vi "Set up rotary stage.vi"(8 "error in (no error)":errorcluster, 11 "AOTF in":refnum<class "AOTF.lvclass">) -> (0 "error out":errorcluster, 3 "AOTF out":refnum<class "AOTF.lvclass">)   [LabVIEW 2012, in "AOTF.lvclass"]
uses:
  AOTF.lvclass
  AOTF.lvclass/AOTF.ctl
panel:
  in  "MG17Motor":refnum<k7>(container)
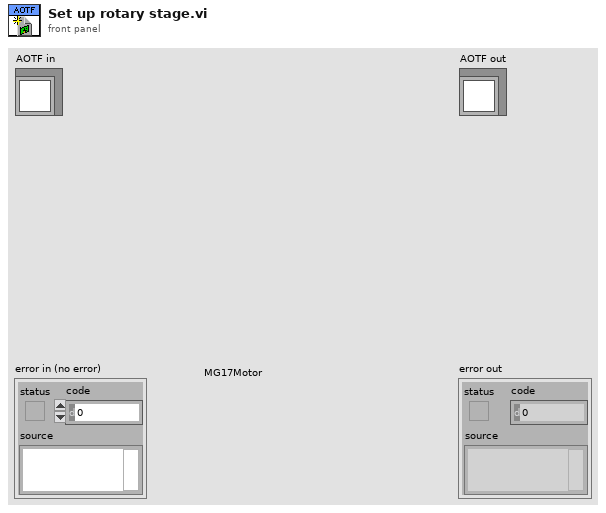
[diagram p1: front panel]
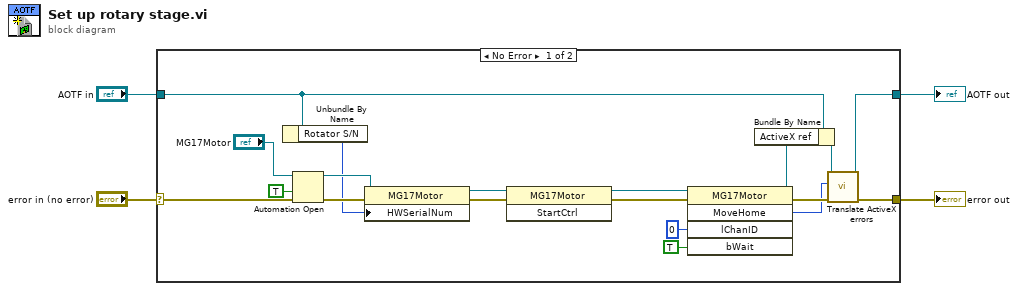
[diagram p0: block diagram]
diagram:
  n1 = case shown="No Error" "error in (no error)" {
    selector: "error in (no error)" -> [w21 w25]
    tunnel: [w7 w25] -> w3
    tunnel: [w9 w24] -> w1
    tunnel: "AOTF in" -> [w16 w24]
    frame No Error {
      n2 = Unbundle By Name(w16) -> ("Rotator S/N"=w19:i32)
      n3 = Automation Open(error in (no error)=w21, Automation Refnum="MG17Motor", 9:TRUE ("open new instance (false)")) -> (Automation Refnum=w22:refnum<k7>, error out=w20:errorcluster)  [unwired: 1 in]
      n4 = property class="MG17Motor"(reference=w22, error in=w20, "HWSerialNum"=w19) -> (reference out=w18:refnum<k7>, error out=w17:errorcluster)
      n5 = invoke class="MG17Motor" method="StartCtrl"(reference=w18, error in=w17) -> (reference out=w15:refnum<k7>, error out=w13:errorcluster)  [unwired: 1 in, 1 out]
      n6 = invoke class="MG17Motor" method="MoveHome"(reference=w15, error in=w13, "lChanID"=0, "bWait"=TRUE) -> (reference out=w14:refnum<k7>, error out=w8:errorcluster, "MoveHome"=w6:i32)  [unwired: 1 in, 2 out]
      n7 = Bundle By Name(cluster=w16, "ActiveX ref"=w14) -> (w10:refnum<class "AOTF.lvclass">)
      n8 = call-dynamic "Translate ActiveX errors.vi"("error in (no error)"=w8, "ActiveX return"=w6, "AOTF in"=w10) -> ("error out"=w7:errorcluster, "AOTF out"=w9:refnum<class "AOTF.lvclass">)  [unwired: 7 in]
    }
    frame Error {
    }
  }
  "error out" <- w3
  "AOTF out" <- w1
